vi "init.vi"(8 "error in (no error)":errorcluster, 11 "CompactRIO in":refnum<class "CompactRIO.lvclass">) -> (0 "error out":errorcluster, 3 "CompactRIO out":refnum<class "CompactRIO.lvclass">)   [LabVIEW 2015, in "CompactRIO.lvclass"]
doc: "Initizializes object."
uses:
  CompactRIO.lvclass
  CompactRIO.lvclass/CompactRIO.ctl
  ComponentTemplateCore/ComponentModel/ComponentModelRT/RIOHandler/IRIOHandler/IRIOHandler.lvclass
  ComponentTemplateCore/ComponentModel/ComponentModelRT/LoopTimer/ILoopTimer/ILoopTimer.lvclass
  ComponentTemplateCore/ComponentModel/ComponentModelRT/IRQHandler/IIRQHandler/IIRQHandler.lvclass
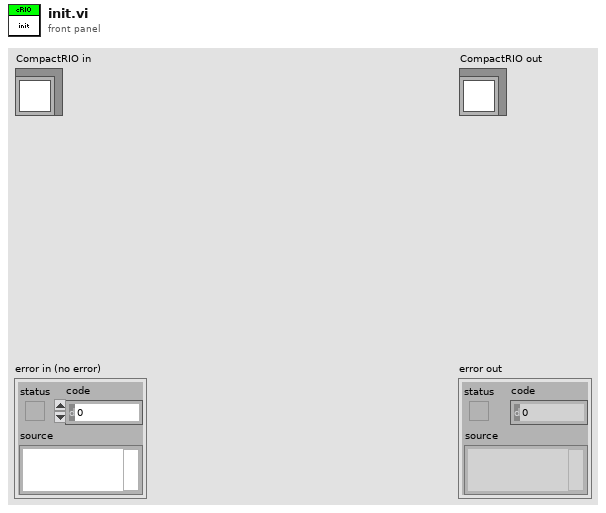
[diagram p1: front panel]
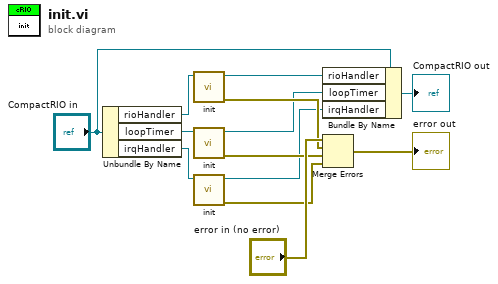
[diagram p0: block diagram]
diagram:
  n1 = Unbundle By Name("CompactRIO in") -> ("rioHandler"=w13:refnum<class "IRIOHandler.lvclass">, "loopTimer"=w6:refnum<class "ILoopTimer.lvclass">, "irqHandler"=w3:refnum<class "IIRQHandler.lvclass">)
  n2 = call-dynamic "init.vi"("IRIOHandler in"=w13) -> ("error out"=w11:errorcluster, "IRIOHandler out"=w9:refnum<class "IRIOHandler.lvclass">)  [unwired: 9 in]
  n3 = call-dynamic "init.vi"("ILoopTimer in"=w6) -> ("error out"=w5:errorcluster, "ILoopTimer out"=w4:refnum<class "ILoopTimer.lvclass">)  [unwired: 9 in]
  n4 = call-dynamic "init.vi"("IIRQHandler in"=w3) -> ("error out"=w1:errorcluster, "IIRQHandler out"=w2:refnum<class "IIRQHandler.lvclass">)  [unwired: 9 in]
  n5 = Bundle By Name(cluster="CompactRIO in", "rioHandler"=w9, "loopTimer"=w4, "irqHandler"=w2) -> (→"CompactRIO out":refnum<class "CompactRIO.lvclass">)
  n6 = Merge Errors("error in (no error)", w11, w5, w1) -> (→"error out":errorcluster)
